vi "PAN_DBS.vi"(7 "Cmd":string, 11 "error in":errorcluster) -> (4 "ImmedReplyString":string, 15 "error out":errorcluster)   [LabVIEW 2016]
uses:
  Modules/DBSHAND/private/vis/DatabaseHand_Element_Get(string).vi
  Modules/DBSHAND/private/vis/DatabaseHand_Element_Set(string).vi
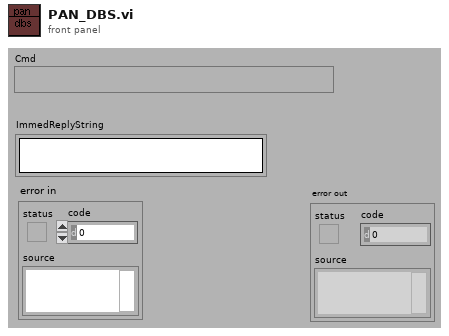
[diagram p1: front panel]
types:
  T1 = typedef "DatabaseHand_RefNum.ctl" = refnum<vi>
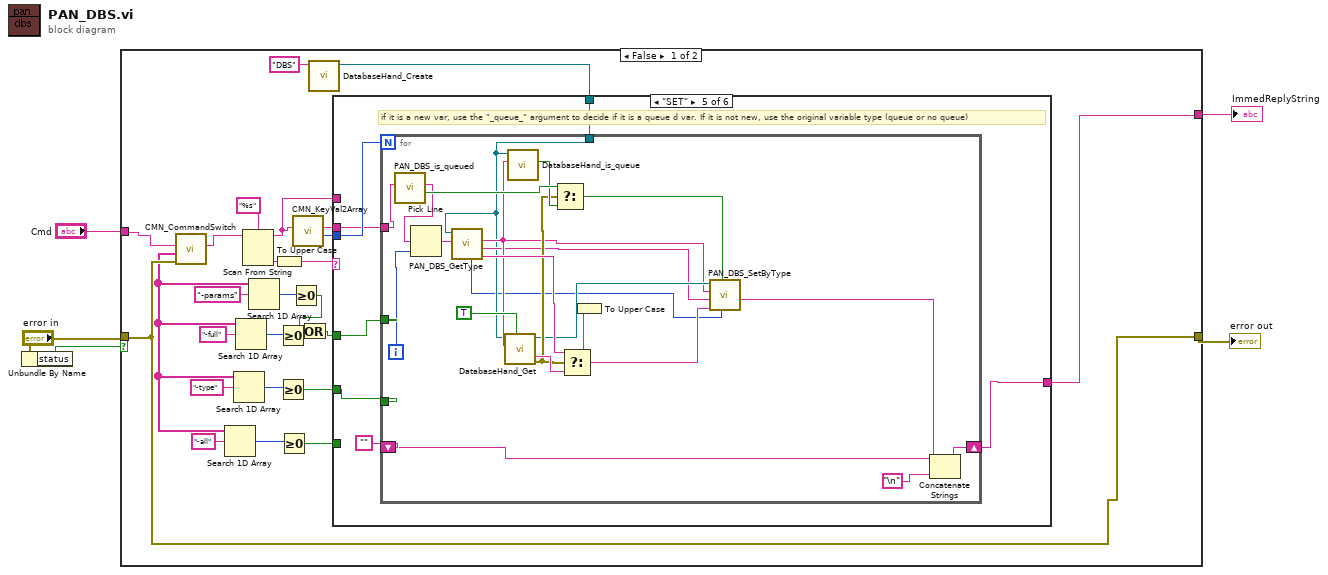
[diagram p0: block diagram]
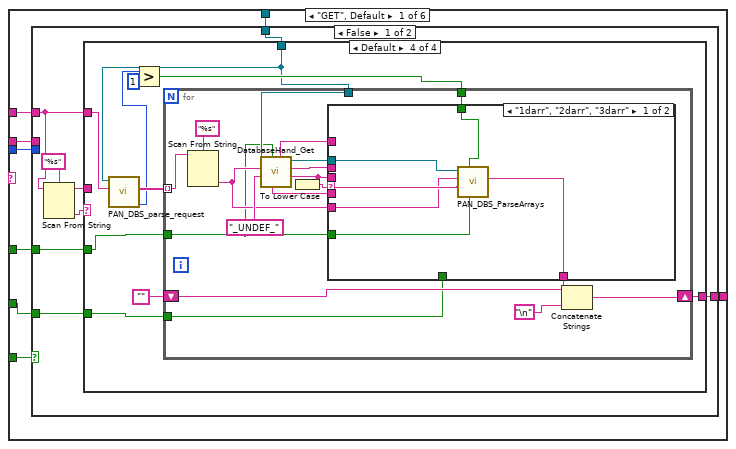
[diagram p2: hidden frame]
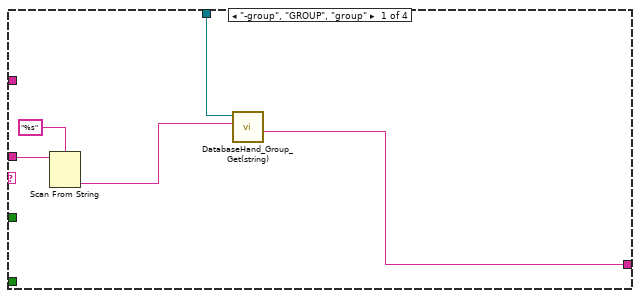
[diagram p3: hidden frame]
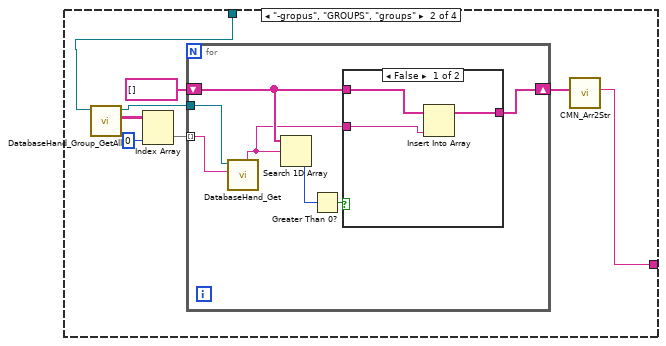
[diagram p4: hidden frame]
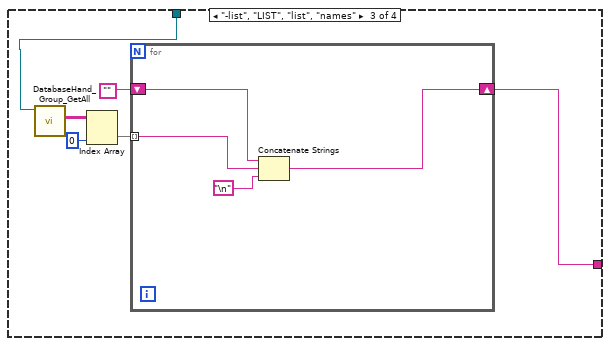
[diagram p6: hidden frame]
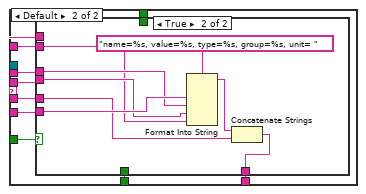
[diagram p7: hidden frame]
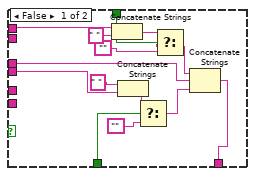
[diagram p8: hidden frame]
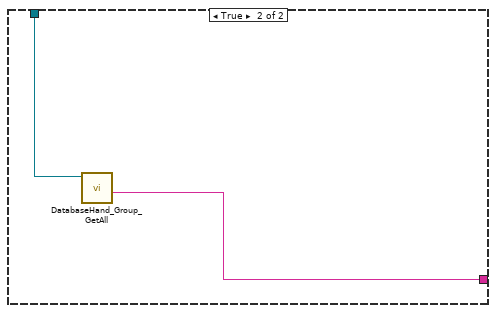
[diagram p9: hidden frame]
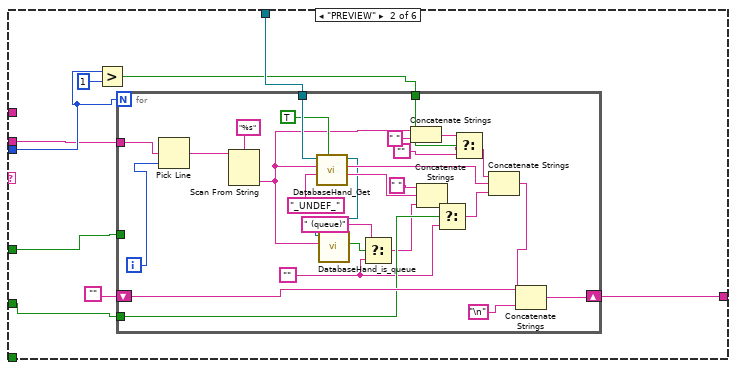
[diagram p10: hidden frame]
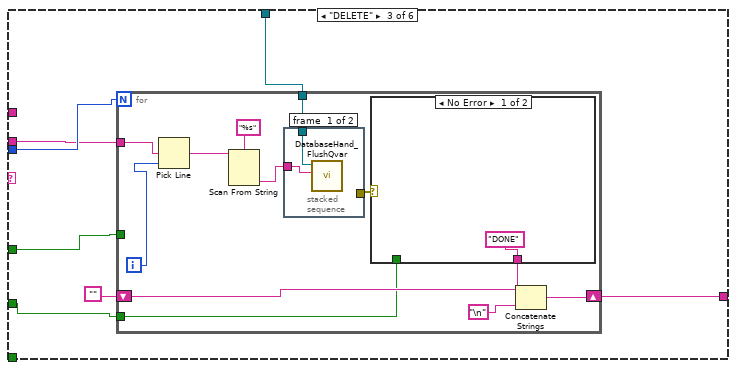
[diagram p11: hidden frame]
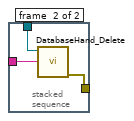
[diagram p12: hidden frame]
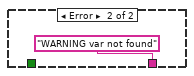
[diagram p13: hidden frame]
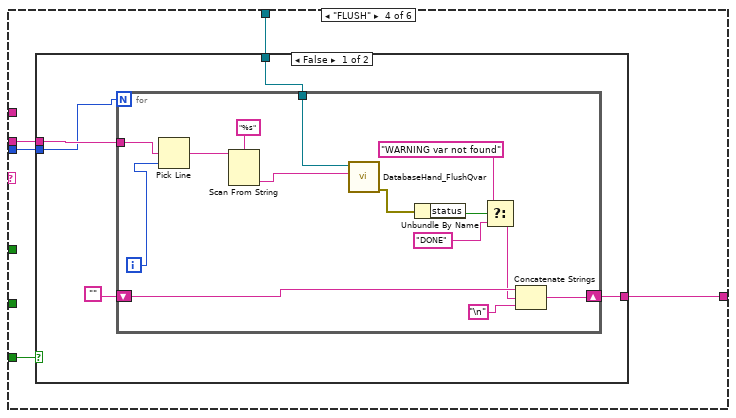
[diagram p14: hidden frame]
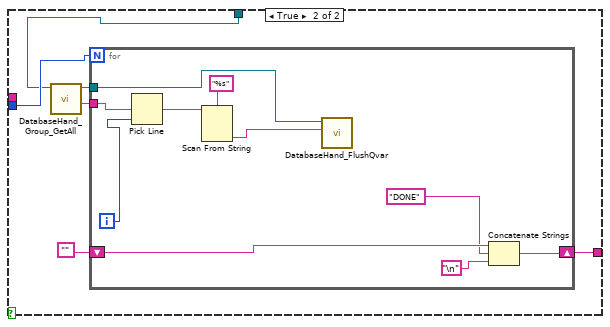
[diagram p15: hidden frame]
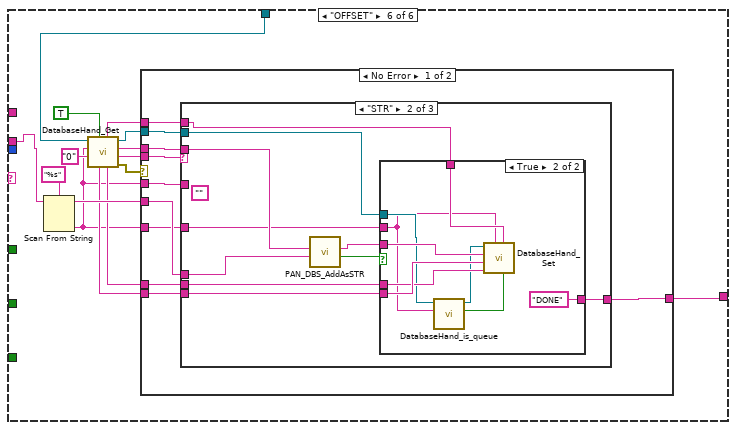
[diagram p16: hidden frame]
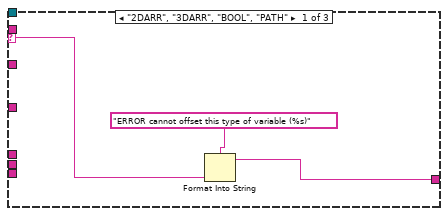
[diagram p17: hidden frame]
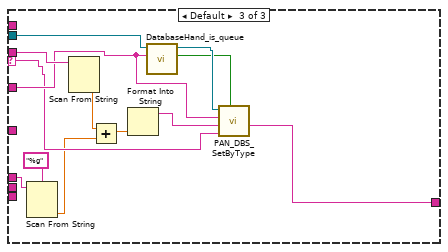
[diagram p19: hidden frame]
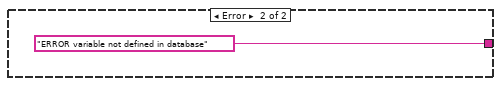
[diagram p20: hidden frame]
diagram:
  n1 = Unbundle By Name("error in") -> ("status"=w3:bool)
  n2 = case shown="False" w3 {
    tunnel: "error in" -> [w18 w343]
    tunnel: [w18 w343] -> w1
    tunnel: [w19 ""] -> w5
    tunnel: "Cmd" -> [w28 _]
    frame False {
      n3 = call "CMN_CommandSwitch.vi"("error in (no error)"=w18, "command in"=w28) -> ("swhitches"=w9:string[], "command out"=w25:string)  [unwired: 8 out]
      n4 = Search 1D Array(1D array=w9, element="-all") -> (index of element=w13:i32)  [unwired: 1 out]
      n5 = Search 1D Array(1D array=w9, element="-type") -> (index of element=w16:i32)  [unwired: 1 out]
      n6 = Search 1D Array(1D array=w9, element="-full") -> (index of element=w21:i32)  [unwired: 1 out]
      n7 = Scan From String(format string="%s" ("Format String"), input string=w25) -> (remaining string=w6:string, output 1=w31:string)  [unwired: 2 in, 3 out]
      n8 = Search 1D Array(1D array=w9, element="-params") -> (index of element=w10:i32)  [unwired: 1 out]
      n9 = To Upper Case(1:w31) -> (0:w29:string)
      n10 = Greater Or Equal To 0?(x=w21) -> (x >= 0?=w20:bool)
      n11 = Greater Or Equal To 0?(x=w16) -> (x >= 0?=w15:bool)
      n12 = Greater Or Equal To 0?(x=w13) -> (x >= 0?=w12:bool)
      n13 = Greater Or Equal To 0?(x=w10) -> (x >= 0?=w7:bool)
      n14 = call "CMN_KeyVal2Array.vi"("command in"=w6) -> ("number of commands"=w23:i32, "commands out"=w24:string)  [unwired: 2 in, 6 out]
      n15 = Or(x=w7, y=w20) -> (x .or. y?=w8:bool)
      n16 = call "DatabaseHand_Create.vi"("Name"="DBS") -> ("Database RefNum out"=w26:T1)  [unwired: 1 in, 9 out]
      n17 = case shown="\"SET\"" w29 {
        tunnel: w26 -> [w37 w155 w190 w214 w256 w294]
        tunnel: w24 -> [w38 w156 w191 w215 w257 w289]
        tunnel: w23 -> [w39 w157 w192 w216 w258 _]
        tunnel: w8 -> [w36 w154 w189 _ w255 _]
        tunnel: [w35 w153 w188 w213 w252 w292] -> w19
        tunnel: w15 -> [w34 w152 w187 _ w254 _]
        tunnel: w12 -> [w33 _ _ w212 _ _]
        tunnel: w6 -> [w32 _ _ _ _ _]
        frame "GET", Default {
          n18 = case shown="False" w33 {
            tunnel: w39 -> [_ _]
            tunnel: w38 -> [_ _]
            tunnel: w37 -> [w44 w148]
            tunnel: w36 -> [w47 _]
            tunnel: [w46 w147] -> w35
            tunnel: w34 -> [w45 _]
            tunnel: w32 -> [w43 _]
            frame False {
              n19 = Scan From String(format string="%s", input string=w43) -> (remaining string=w40:string, output 1=w41:string)  [unwired: 2 in, 3 out]
              n20 = case shown="Default" w41 {
                tunnel: w47 -> [_ _ _ w91]
                tunnel: [w48 w54 w73 w89] -> w46
                tunnel: w45 -> [_ _ _ w88]
                tunnel: w43 -> [_ _ _ w83]
                tunnel: w44 -> [w52 w60 w77 w82]
                tunnel: w40 -> [w51 _ _ _]
                frame "-group", "GROUP", "group" {
                  n21 = Scan From String(format string="%s", input string=w51) -> (output 1=w49:string)  [unwired: 2 in, 4 out]
                  n22 = call "DatabaseHand_Group_Get(string).vi"("group"=w49, "Database RefNum in"=w52) -> ("group string"=w48:string)  [unwired: 1 in, 8 out]
                }
                frame "-gropus", "GROUPS", "groups" {
                  n23 = call "DatabaseHand_Group_GetAll.vi"("Database RefNum in"=w60) -> ("database array"=w59:string[][], "Database RefNum out"=w53:T1)  [unwired: 1 in, 8 out]
                  n24 = Index Array(array=w59, index (col)=0 ("disabled index (col)")) -> (element=w57:string[])  [unwired: 1 in]
                  n25 = for {
                    tunnel: w57 -> [w62] mode=indexing
                    shift-right: [w65] -> w55
                    shift-left: string[] [] -> [w64]
                    tunnel: w53 -> [w63]
                    n26 = call-poly "DatabaseHand_Get.vi"("name"=w62, "Database RefNum in"=w63) -> ("group"=w61:string)  [unwired: 3 in, 6 out]
                    n27 = Search 1D Array(1D array=w64, element=w61) -> (index of element=w67:i32)  [unwired: 1 out]
                    n28 = Greater Than 0?(x=w67) -> (x > 0?=w66:bool)
                    n29 = case shown="False" w66 {
                      tunnel: w61 -> [w70 _]
                      tunnel: [w69 w71] -> w65
                      tunnel: w64 -> [w68 w71]
                      frame False {
                        n30 = Insert Into Array(array=w68, new element=w70) -> (w69:string[])  [unwired: 1 in]
                      }
                      frame True {
                      }
                    }
                  }
                  n31 = call "CMN_Arr2Str.vi"("Array in"=w55) -> ("string out"=w54:string)  [unwired: 10 out]
                }
                frame "-list", "LIST", "list", "names" {
                  n32 = call "DatabaseHand_Group_GetAll.vi"("Database RefNum in"=w77) -> ("database array"=w76:string[][])  [unwired: 1 in, 9 out]
                  n33 = Index Array(array=w76, index (col)=0 ("disabled index (col)")) -> (element=w74:string[])  [unwired: 1 in]
                  n34 = for {
                    tunnel: w74 -> [w79] mode=indexing
                    shift-right: [w81] -> w73
                    shift-left: "" -> [w80]
                    n35 = Concatenate Strings(w80, w79, "\n") -> (w81:string)
                  }
                }
                frame Default {
                  n36 = call "PAN_DBS_parse_request.vi"("desired point"=w83, "Database RefNum in"=w82) -> ("number of points"=w84:i32, "names"=w85:string[])  [unwired: 1 in, 7 out]
                  n37 = Greater?(x=w84, y=1) -> (0:w86:bool)
                  n38 = for {
                    tunnel: w82 -> [w108]
                    tunnel: w91 -> [w97]
                    shift-right: [w104] -> w89
                    shift-left: "" -> [w103]
                    tunnel: w88 -> [w101]
                    tunnel: w86 -> [w98]
                    tunnel: w85 -> [w95] mode=indexing
                    n39 = Scan From String(format string="%s", input string=w95) -> (output 1=w99:string)  [unwired: 2 in, 4 out]
                    n40 = call-poly "DatabaseHand_Get.vi"("nd queue"=w97, "default value"="_UNDEF_", "name"=w99, "Database RefNum in"=w108) -> ("type"=w94:string, "value"=w107:string, "Database RefNum out"=w92:T1, "group"=w106:string, "unit"=w96:string)  [unwired: 1 in, 2 out]
                    n41 = To Lower Case(string=w94) -> (all lower case string=w93:string)
                    n42 = case shown="\"1darr\", \"2darr\", \"3darr\"" w93 {
                      selector: w93 -> [w113 _]
                      tunnel: w107 -> [_ w124]
                      tunnel: w106 -> [_ w123]
                      tunnel: [w115 w122] -> w105
                      tunnel: w101 -> [_ w121]
                      tunnel: w99 -> [w112 w120]
                      tunnel: w98 -> [w110 w119]
                      tunnel: w97 -> [w111 w118]
                      tunnel: w96 -> [_ w117]
                      tunnel: w94 -> [_ w116]
                      tunnel: w92 -> [w114 _]
                      frame "1darr", "2darr", "3darr" {
                        n43 = call "PAN_DBS_ParseArrays.vi"("full"=w111, "name_only"=w110, "type"=w113, "name"=w112, "Database RefNum in"=w114) -> ("str out"=w115:string)  [unwired: 6 out]
                      }
                      frame Default {
                        n44 = case shown="True" w118 {
                          tunnel: w124 -> [w138 w145]
                          tunnel: w116 -> [w132 w144]
                          tunnel: w120 -> [_ w146]
                          tunnel: w123 -> [_ w143]
                          tunnel: [w134 w141] -> w122
                          tunnel: w121 -> [w137 _]
                          tunnel: w120 -> [w127 _]
                          tunnel: w119 -> [w129 _]
                          tunnel: w117 -> [_ w142]
                          frame False {
                            n45 = Concatenate Strings(w127, " " ("string")) -> (w126:string)
                            n46 = Concatenate Strings(" " ("string"), w132) -> (w131:string)
                            n47 = Select(t=w131, s=w137, f="") -> (s? t:f=w135:string)
                            n48 = Select(t=w126, s=w129, f="") -> (s? t:f=w128:string)
                            n49 = Concatenate Strings(w128, w138, w135) -> (w134:string)
                          }
                          frame True {
                            n50 = Format Into String(format string="name=%s, value=%s, type=%s, group=%s, unit= ", w146, w145, w144, w143) -> (resulting string=w139:string)  [unwired: 2 in, 1 out]
                            n51 = Concatenate Strings(w139, w142) -> (w141:string)
                          }
                        }
                      }
                    }
                    n52 = Concatenate Strings(w103, w105, "\n") -> (w104:string)
                  }
                }
              }
            }
            frame True {
              n53 = call "DatabaseHand_Group_GetAll.vi"("Database RefNum in"=w148) -> ("database string string"=w147:string)  [unwired: 1 in, 9 out]
            }
          }
        }
        frame "PREVIEW" {
          n54 = Greater?(x=w157, y=1) -> (0:w149:bool)
          n55 = for {
            N: w157 -> [_]
            tunnel: w156 -> [w184]
            tunnel: w155 -> [w181]
            tunnel: w154 -> [_]
            shift-right: [w177] -> w153
            shift-left: "" -> [w176]
            tunnel: w152 -> [w174]
            tunnel: w149 -> [w172]
            i -> [w183]
            w160 = ""
            n56 = Pick Line(multi-line string=w184, line index=w183) -> (output string=w182:string)  [unwired: 1 out]
            n57 = Scan From String(format string="%s", input string=w182) -> (output 1=w163:string)  [unwired: 2 in, 4 out]
            n58 = call-poly "DatabaseHand_Get.vi"("nd queue"=TRUE, "default value"="_UNDEF_", "name"=w163, "Database RefNum in"=w181) -> ("type"=w179:string, "value"=w180:string, "Database RefNum out"=w162:T1)  [unwired: 1 in, 4 out]
            n59 = call "DatabaseHand_is_queue.vi"("name"=w163, "Database RefNum in"=w162) -> ("queue?"=w161:bool)  [unwired: 1 in, 8 out]
            n60 = Select(t=" (queue)", s=w161, f=w160) -> (s? t:f=w158:string)
            n61 = Concatenate Strings(w163, " " ("string")) -> (w165:string)
            n62 = Concatenate Strings(" " ("string"), w179, w158) -> (w168:string)
            n63 = Select(t=w168, s=w174, f=w160) -> (s? t:f=w170:string)
            n64 = Select(t=w165, s=w172, f="") -> (s? t:f=w166:string)
            n65 = Concatenate Strings(w166, w180, w170) -> (w178:string)
            n66 = Concatenate Strings(w176, w178, "\n") -> (w177:string)
          }
        }
        frame "DELETE" {
          n67 = for {
            N: w192 -> [_]
            tunnel: w191 -> [w203]
            tunnel: w190 -> [w194]
            tunnel: w189 -> [_]
            shift-right: [w199] -> w188
            shift-left: "" -> [w198]
            tunnel: w187 -> [w196]
            i -> [w202]
            n68 = Pick Line(multi-line string=w203, line index=w202) -> (output string=w201:string)  [unwired: 1 out]
            n69 = Scan From String(format string="%s", input string=w201) -> (output 1=w193:string)  [unwired: 2 in, 4 out]
            n70 = stacked-sequence {
              tunnel: [_ w209] -> w195
              tunnel: w194 -> [w206 w208]
              tunnel: w193 -> [w205 w207]
              frame #0 {
                n71 = call "DatabaseHand_FlushQvar.vi"("name"=w205, "Database RefNum In"=w206) -> ()  [unwired: 1 in, 9 out]
              }
              frame #1 {
                n72 = call "DatabaseHand_Delete.vi"("name"=w207, "Database RefNum in"=w208) -> ("error out"=w209:errorcluster)  [unwired: 1 in, 8 out]
              }
            }
            n73 = case shown="No Error" w195 {
              tunnel: ["DONE" "WARNING var not found"] -> w200
              tunnel: w196 -> [_ _]
              frame No Error {
              }
              frame Error {
              }
            }
            n74 = Concatenate Strings(w198, w200, "\n") -> (w199:string)
          }
        }
        frame "FLUSH" {
          n75 = case shown="False" w212 {
            tunnel: w216 -> [w217 w239]
            tunnel: w215 -> [w221 _]
            tunnel: w214 -> [w220 w238]
            tunnel: [w218 w240] -> w213
            frame False {
              n76 = for {
                N: w217 -> [_]
                tunnel: w221 -> [w234]
                tunnel: w220 -> [w228]
                shift-right: [w231] -> w218
                shift-left: "" -> [w230]
                i -> [w233]
                n77 = Pick Line(multi-line string=w234, line index=w233) -> (output string=w232:string)  [unwired: 1 out]
                n78 = Scan From String(format string="%s", input string=w232) -> (output 1=w227:string)  [unwired: 2 in, 4 out]
                n79 = call "DatabaseHand_FlushQvar.vi"("name"=w227, "Database RefNum In"=w228) -> ("error out"=w226:errorcluster)  [unwired: 1 in, 8 out]
                n80 = Unbundle By Name(w226) -> ("status"=w225:bool)
                n81 = Select(t="WARNING var not found", s=w225, f="DONE") -> (s? t:f=w223:string)
                n82 = Concatenate Strings(w230, w223, "\n") -> (w231:string)
              }
            }
            frame True {
              n83 = call "DatabaseHand_Group_GetAll.vi"("Database RefNum in"=w238) -> ("database string string"=w236:string, "Database RefNum out"=w237:T1)  [unwired: 1 in, 8 out]
              n84 = for {
                N: w239 -> [_]
                shift-right: [w248] -> w240
                shift-left: "" -> [w247]
                tunnel: w237 -> [w244]
                tunnel: w236 -> [w243]
                i -> [w250]
                n85 = Pick Line(multi-line string=w243, line index=w250) -> (output string=w249:string)  [unwired: 1 out]
                n86 = Scan From String(format string="%s", input string=w249) -> (output 1=w245:string)  [unwired: 2 in, 4 out]
                n87 = call "DatabaseHand_FlushQvar.vi"("name"=w245, "Database RefNum In"=w244) -> ()  [unwired: 1 in, 9 out]
                n88 = Concatenate Strings(w247, "DONE", "\n") -> (w248:string)
              }
            }
          }
        }
        frame "SET" {
          # "if it is a new var, use the \"_queue_\" argument to decide if it is a queue d var. If it is not new, use the original variable type (queue or no queue)"
          n89 = for {
            N: w258 -> [_]
            tunnel: w257 -> [w274]
            tunnel: w256 -> [w260]
            tunnel: w255 -> [_]
            tunnel: w254 -> [_]
            shift-right: [w277] -> w252
            shift-left: "" -> [w276]
            i -> [w279]
            n90 = call "PAN_DBS_is_queued.vi"("args in"=w274) -> ("queue?"=w272:bool, "args out"=w261:string)  [unwired: 9 out]
            n91 = Pick Line(multi-line string=w261, line index=w279) -> (output string=w269:string)  [unwired: 1 out]
            n92 = call "PAN_DBS_GetType.vi"("cmd in"=w269, "Database RefNum out"=w260) -> ("datatype"=w270:string, "value"=w263:string, "name"=w264:string, "precision"=w259:i32)  [unwired: 6 out]
            n93 = call-poly "DatabaseHand_Get.vi"("nd queue"=TRUE, "name"=w264, "Database RefNum in"=w260) -> ("error out"=w268:errorcluster, "type"=w275:string, "Database RefNum out"=w267:T1)  [unwired: 2 in, 4 out]
            n94 = call "DatabaseHand_is_queue.vi"("name"=w264, "Database RefNum in"=w260) -> ("queue?"=w271:bool)  [unwired: 1 in, 8 out]
            n95 = Select(t=w272, s=w268, f=w271) -> (s? t:f=w266:bool)
            n96 = Select(t=w270, s=w268, f=w275) -> (s? t:f=w262:string)
            n97 = To Upper Case(1:w262) -> ()  [unwired: 1 out]
            n98 = call "PAN_DBS_SetByType.vi"("precision"=w259, "queue?"=w266, "type"=w262, "value"=w263, "name"=w264, "Database RefNum"=w267) -> ("response"=w265:string)  [unwired: 5 out]
            n99 = Concatenate Strings(w276, w265, "\n") -> (w277:string)
          }
        }
        frame "OFFSET" {
          n100 = Scan From String(format string="%s", input string=w289) -> (remaining string=w288:string, output 1=w280:string)  [unwired: 2 in, 3 out]
          n101 = call-poly "DatabaseHand_Get.vi"("nd queue"=TRUE, "default value"="0", "name"=w280, "Database RefNum in"=w294) -> ("error out"=w293:errorcluster, "type"=w291:string, "value"=w287:string, "Database RefNum out"=w284:T1, "permissions"=w281:string, "group"=w283:string, "unit"=w282:string)  [unwired: 1 in]
          n102 = case shown="No Error" w293 {
            tunnel: [w300 "ERROR variable not defined in database" ("database string string")] -> w292
            tunnel: w291 -> [w304 _]
            tunnel: w288 -> [w299 _]
            tunnel: w287 -> [w303 _]
            tunnel: w284 -> [w302 _]
            tunnel: w280 -> [w301 _]
            tunnel: w283 -> [w298 _]
            tunnel: w282 -> [w297 _]
            tunnel: w281 -> [w296 _]
            tunnel: w280 -> [w295 _]
            frame No Error {
              n103 = case shown="\"STR\"" w304 {
                selector: w304 -> [w306 _ w332]
                tunnel: w303 -> [_ w317 w340]
                tunnel: w302 -> [_ w315 w337]
                tunnel: w301 -> [_ _ w334]
                tunnel: [w307 w309 w331] -> w300
                tunnel: w299 -> [_ w314 w329]
                tunnel: w298 -> [_ w312 _]
                tunnel: w297 -> [_ w311 _]
                tunnel: w296 -> [_ w310 _]
                tunnel: w295 -> [_ w308 _]
                frame "2DARR", "3DARR", "BOOL", "PATH" {
                  n104 = Format Into String(format string="ERROR cannot offset this type of variable (%s)" ("response"), w306) -> (resulting string=w307:string)  [unwired: 2 in, 1 out]
                }
                frame "STR" {
                  (unwired) ""
                  n105 = call "PAN_DBS_AddAsSTR.vi"("offset"=w314, "ini value"=w317) -> ("ok?"=w316:bool, "value out"=w313:string)  [unwired: 8 out]
                  n106 = case shown="True" w316 {
                    tunnel: w315 -> [_ w323]
                    tunnel: w313 -> [w318 w327]
                    tunnel: w312 -> [_ w326]
                    tunnel: w311 -> [_ w325]
                    tunnel: w310 -> [_ w324]
                    tunnel: [w318 "DONE" ("value out")] -> w309
                    tunnel: w308 -> [_ w319]
                    frame False {
                    }
                    frame True {
                      n107 = call "DatabaseHand_is_queue.vi"("name"=w319, "Database RefNum in"=w323) -> ("queue?"=w321:bool, "Database RefNum out"=w322:T1)  [unwired: 1 in, 7 out]
                      n108 = call-poly "DatabaseHand_Set.vi"("enqueue? (F)"=w321, "group"=w326, "permissions"=w324, "name"=w319, "unit"=w325, "value"=w327, "Database RefNum in"=w322) -> ()  [unwired: 1 in, 4 out]
                    }
                  }
                }
                frame Default {
                  n109 = Scan From String(format string="%g", input string=w329) -> (output 1=w328:dbl)  [unwired: 2 in, 4 out]
                  n110 = Scan From String(input string=w340) -> (output 1=w339:dbl)  [unwired: 3 in, 4 out]
                  n111 = Add(x=w339, y=w328) -> (x+y=w338:dbl)
                  n112 = Format Into String(w338) -> (resulting string=w333:string)  [unwired: 3 in, 1 out]
                  n113 = call "DatabaseHand_is_queue.vi"("name"=w334, "Database RefNum in"=w337) -> ("queue?"=w335:bool, "Database RefNum out"=w336:T1)  [unwired: 1 in, 7 out]
                  n114 = call "PAN_DBS_SetByType.vi"("queue?"=w335, "type"=w332, "value"=w333, "name"=w334, "Database RefNum"=w336) -> ("response"=w331:string)  [unwired: 1 in, 5 out]
                }
              }
            }
            frame Error {
            }
          }
        }
      }
    }
    frame True {
    }
  }
  "error out" <- w1
  "ImmedReplyString" <- w5
